vi "advent_4.vi"() -> ()   [LabVIEW 2021]
uses:
  <vilib>/Utility/file.llb/Read Delimited Spreadsheet (string).vi
  <vilib>/Utility/file.llb/Read Delimited Spreadsheet (I64).vi
panel:
  out "array w/ subset deleted":string[][](array[string])
  out "all rows 2":string[][](array[string])
  out "final value":i32
  out "last number called":u8
  out "sum of unmarked":i32
  out "all rows":string[](array[string])
  out "size(s)":i32
  out "final bingo call":i32
  out "Book Number":i32
  out "Array":bool[][][](array[boolean])
  out "subarray 3":i32[][](array[numeric])
  out "card":bool[][](array[boolean])
  out "initialized array":bool[][][](array[boolean])
  out "Array 2":i32[][][](array[numeric])
  out "subarray":string[](array[string])
  out "first row":i64[](array[numeric])
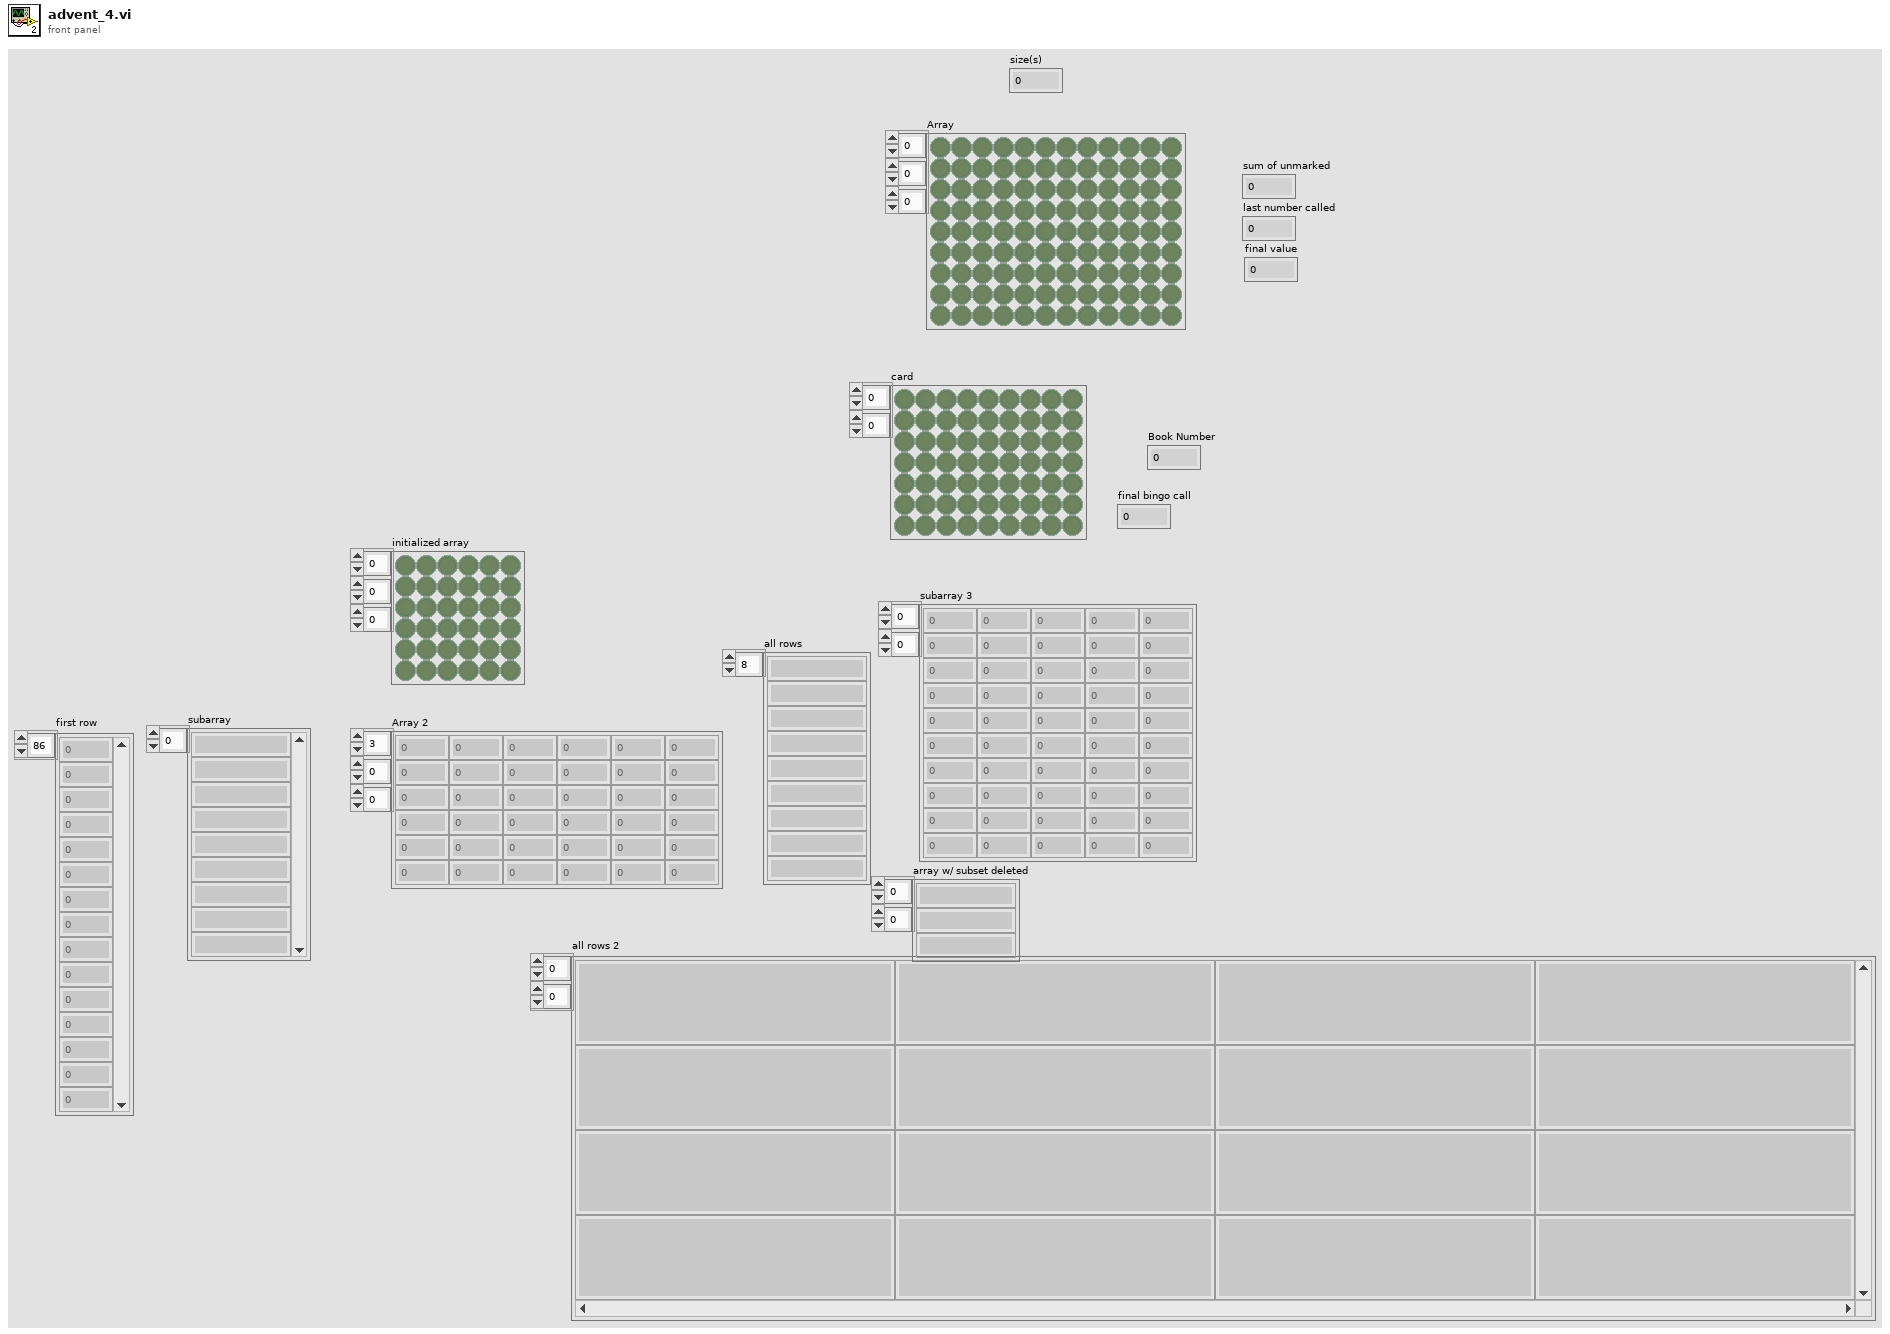
[diagram p1: front panel]
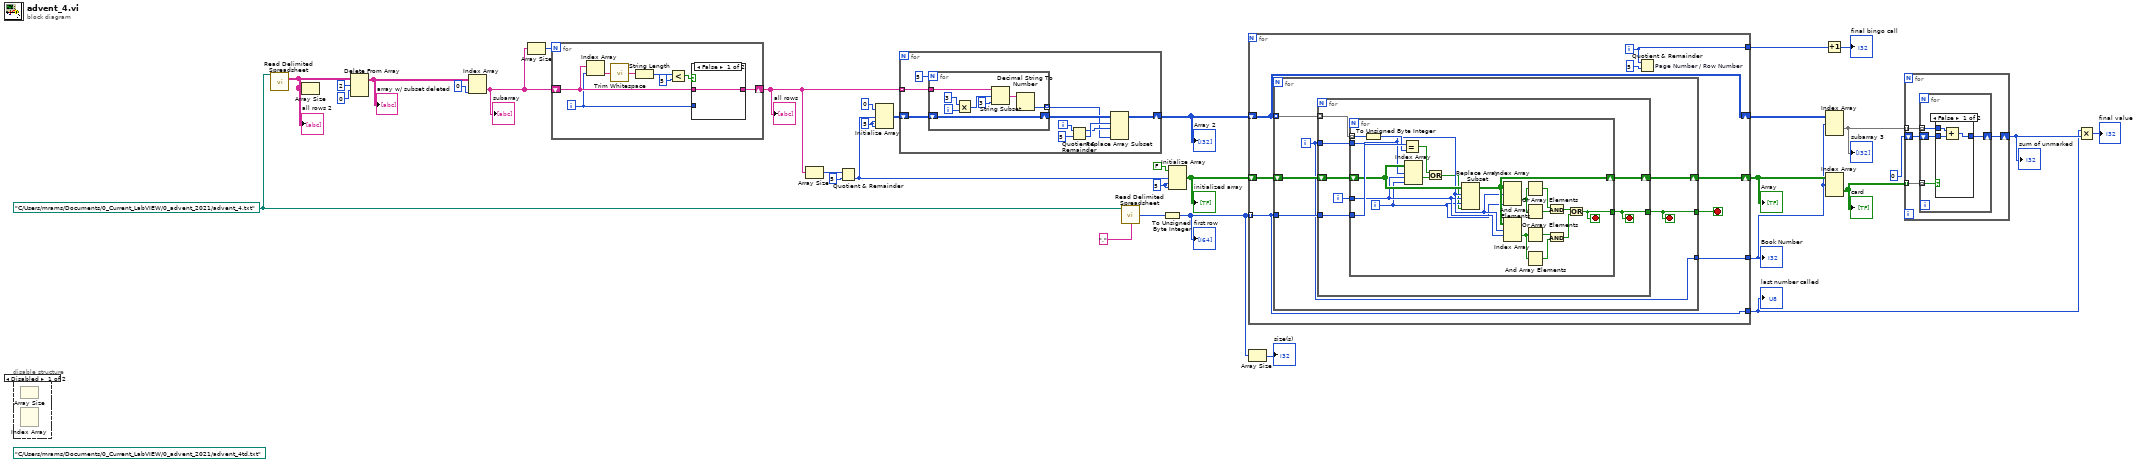
[diagram p0: block diagram]
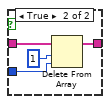
[diagram p3: hidden frame]
diagram:
  w1 = path "C:/Users/mrams/Documents/0_Current_LabVIEW/0_advent_2021/advent_4.txt" ("file path (dialog if empty)")
  w21 = 5 ("dimension size")
  w22 = 5 ("dimension size")
  (unwired) path "C:/Users/mrams/Documents/0_Current_LabVIEW/0_advent_2021/advent_4td.txt" ("file path (dialog if empty)")
  n1 = disable-structure shown="Disabled" {
    frame Disabled {
      n2 = Array Size() -> ()  [unwired: 1 in, 1 out]
      n3 = Index Array() -> ()  [unwired: 3 in, 1 out]
    }
    frame Enabled {
    }
  }
  n4 = call-poly <vilib>:"Read Delimited Spreadsheet.vi"("file path (dialog if empty)"=w1) -> ("all rows"=w2:string[][])  [unwired: 9 in, 5 out]
  "all rows 2" <- w2
  n5 = Array Size(array=w2) -> ()  [unwired: 1 out]
  n6 = Delete From Array(array=w2, length=2, index (row)=0) -> (array with subset deleted=w31:string[][])  [unwired: 1 in, 1 out]
  "array w/ subset deleted" <- w31
  n7 = Index Array(array=w31, index (col)=0 ("disabled index (col)")) -> (element=w24:string[])  [unwired: 1 in]
  "subarray" <- w24
  n8 = Array Size(array=w24) -> (size(s)=w23:i32)
  n9 = for {
    N: w23 -> [_]
    shift-right: [w35] -> w27
    shift-left: w24 -> [w42]
    i -> [w41]
    n10 = Index Array(array=w42, index=w41) -> (element=w40:string)
    n11 = call <vilib>:"Trim Whitespace.vi"("string"=w40) -> ("trimmed string"=w39:string)  [unwired: 1 in]
    n12 = String Length(string=w39) -> (length=w38:i32)
    n13 = Less?(x=w38, y=5) -> (x < y?=w36:bool)
    n14 = case shown="False" w36 {
      tunnel: w42 -> [w43 w47]
      tunnel: w41 -> [_ w46]
      tunnel: [w43 w44] -> w35
      frame False {
      }
      frame True {
        n15 = Delete From Array(array=w47, length=1, index=w46) -> (array with subset deleted=w44:string[])  [unwired: 1 out]
      }
    }
  }
  "all rows" <- w27
  n16 = Array Size(array=w27) -> (size(s)=w26:i32)
  n17 = Quotient & Remainder(x=w26, y=5) -> (floor(x/y)=w19:i32)  [unwired: 1 out]
  n18 = Initialize Array(u8 0, w19, w22, w22) -> (w28:u8[][][])
  n19 = for {
    tunnel: w27 -> [w57] mode=indexing
    shift-right: [w54] -> w17
    shift-left: w28 -> [w56]
    i -> [w52]
    n20 = for {
      N: 5 -> [_]
      tunnel: w57 -> [w65]
      tunnel: [w61] -> w48 mode=indexing
      shift-right: [w60] -> w55
      shift-left: w56 -> [w60]
      i -> [w59]
      n21 = Multiply(x=3, y=w59) -> (x*y=w58:i32)
      n22 = String Subset(string=w65, offset (0)=w58, length (rest)=3 ("length (rest)")) -> (substring=w62:string)
      n23 = Decimal String To Number(string=w62) -> (number=w61:i32)  [unwired: 2 in, 1 out]
    }
    n24 = Quotient & Remainder(x=w52, y=5) -> (x-y*floor(x/y)=w49:i32, floor(x/y)=w50:i32)
    n25 = Replace Array Subset(array=w55, new element=w48, index (dim 0)=w50, index (dim 1)=w49) -> (w54:u8[][][])  [unwired: 1 in]
  }
  "Array 2" <- w17
  n26 = call-poly <vilib>:"Read Delimited Spreadsheet.vi"("file path (dialog if empty)"=w1, "delimiter (\\t)"="," ("delimiter (\\t)")) -> ("first row"=w12:i64[])  [unwired: 8 in, 5 out]
  n27 = To Unsigned Byte Integer(number=w12) -> (unsigned 8bit integer=w9:u8[])
  "first row" <- w9
  n28 = Initialize Array(FALSE, w19, w21, w21) -> (w18:bool[][][])
  "initialized array" <- w18
  n29 = for {
    tunnel: w9 -> [w66] mode=indexing
    shift-right: [w70] -> w16
    shift-left: w18 -> [w73]
    shift-right: [w69] -> w15
    shift-left: w17 -> [w69]
    tunnel: [w67] -> w14
    tunnel: [w68] -> w13
    tunnel: [w66] -> w4
    i -> [w68]
    stop <- w71 stop-if-true
    n30 = for {
      tunnel: w66 -> [w79]
      tunnel: w69 -> [w77] mode=indexing
      shift-right: [w76] -> w70
      shift-left: w73 -> [w78]
      tunnel: [w75] -> w71
      tunnel: [w74] -> w67
      i -> [w74]
      stop <- w75 stop-if-true
      n31 = for {
        tunnel: w79 -> [w84]
        tunnel: w77 -> [w85] mode=indexing
        shift-right: [w82] -> w76
        shift-left: w78 -> [w86]
        tunnel: w74 -> [w83]
        tunnel: [w81] -> w75
        i -> [w80]
        stop <- w81 stop-if-true
        n32 = for {
          tunnel: w85 -> [w105] mode=indexing
          tunnel: w84 -> [w106]
          shift-right: [w104] -> w82
          shift-left: w86 -> [w93]
          tunnel: w83 -> [w92]
          tunnel: w80 -> [w91]
          tunnel: [w103] -> w81
          i -> [w90]
          stop <- w103 stop-if-true
          n33 = To Unsigned Byte Integer(number=w105) -> (unsigned 8bit integer=w94:u8)
          n34 = Equal?(x=w106, y=w94) -> (x = y?=w88:bool)
          n35 = Index Array(array=w93, index (dim 0)=w92, index (dim 1)=w91, index (dim 2)=w90) -> (element=w89:bool)
          n36 = Or(x=w88, y=w89) -> (x .or. y?=w87:bool)
          n37 = Replace Array Subset(array=w93, new element=w87, index (dim 0)=w92, index (dim 1)=w91, index (dim 2)=w90) -> (w104:bool[][][])
          n38 = Index Array(array=w104, index (dim 0)=w92, index (dim 2)=w90) -> (element=w101:bool[])  [unwired: 1 in]
          n39 = Index Array(array=w104, index (dim 0)=w92, index (dim 1)=w91) -> (element=w102:bool[])  [unwired: 1 in]
          n40 = Or Array Elements(Boolean array=w101) -> (logical OR=w98:bool)
          n41 = And Array Elements(Boolean array=w101) -> (logical AND=w97:bool)
          n42 = Or Array Elements(Boolean array=w102) -> (logical OR=w100:bool)
          n43 = And Array Elements(Boolean array=w102) -> (logical AND=w99:bool)
          n44 = And(x=w98, y=w97) -> (x .and. y?=w96:bool)
          n45 = And(x=w100, y=w99) -> (x .and. y?=w95:bool)
          n46 = Or(x=w96, y=w95) -> (x .or. y?=w103:bool)
        }
      }
    }
    n47 = Quotient & Remainder "Page Number / Row Number"(x=w68, y=5) -> ()  [unwired: 2 out]
  }
  "Array" <- w16
  "Book Number" <- w14
  "last number called" <- w4
  n48 = Array Size(array=w9) -> (size(s)=→"size(s)":i32)
  n49 = Increment(x=w13) -> (x+1=→"final bingo call":i32)
  n50 = Index Array(array=w15, index (dim 0)=w14) -> (element=w7:u8[][])  [unwired: 2 in]
  "subarray 3" <- w7
  n51 = Index Array(array=w16, index (dim 0)=w14) -> (element=w8:bool[][])  [unwired: 2 in]
  "card" <- w8
  n52 = for {
    tunnel: w8 -> [w110] mode=indexing
    tunnel: w7 -> [w109] mode=indexing
    shift-right: [w107] -> w5
    shift-left: 0 -> [w108]
    n53 = for {
      tunnel: w110 -> [w114] mode=indexing
      tunnel: w109 -> [w113] mode=indexing
      shift-right: [w111] -> w107
      shift-left: w108 -> [w112]
      n54 = case shown="False" w114 {
        tunnel: w113 -> [w117 _]
        tunnel: w112 -> [w116 w118]
        tunnel: [w115 w118] -> w111
        frame False {
          n55 = Add(x=w117, y=w116) -> (x+y=w115:i32)
        }
        frame True {
        }
      }
    }
  }
  "sum of unmarked" <- w5
  n56 = Multiply(x=w4, y=w5) -> (x*y=→"final value":i32)
